vi "penaltyTactic.vi"(7 "firstCall":bool=TRUE, 8 "error in (no error)":errorcluster, 9 "Game in":refnum<class "Game.lvclass">, 10 "RobotRef":refnum<class "Robot.lvclass">, 11 "PenaltyTactic in":refnum<class "PenaltyTactic.lvclass">) -> (0 "error out":errorcluster, 2 "Robot out":refnum<class "Robot.lvclass">, 3 "PenaltyTactic out":refnum<class "PenaltyTactic.lvclass">)   [LabVIEW 2024, in "PenaltyTactic.lvclass"]
uses:
  PenaltyTactic.lvclass
  C:/Users/as119/OneDrive/Documentos/roboIME/SSL_AI/Tactic_class/Tactic.lvclass
  Robot_class/Robot.lvclass
  C:/Users/as119/OneDrive/Documentos/roboIME/SSL_AI/Object_class/Object.lvclass
  Game_class/Game.lvclass
  Robot_class/tactics.ctl
  Control 2.ctl
  Tactic_class/Tactic.lvclass/Tactic.ctl
  Game_class/Game.lvclass/Game.ctl
  Parameters_class/Parameters.lvclass/Parameters.ctl
  Team_class/Team.lvclass/Team.ctl
  Referee_class/Referee.lvclass/Referee.ctl
  Object_class/Object.lvclass/Object.ctl
  Skillbook_class/Skillbook.lvclass/Skillbook.ctl
  Robot_class/Robot.lvclass/Robot.ctl
  Robot_class/robotKickToStates.ctl
  Events_class/Events.lvclass/Events.ctl
  Ball_class/Ball.lvclass/Ball.ctl
  PenaltyTactic.lvclass/PenaltyTactic.ctl
  <vilib>/numeric/Random Number (Range) U64.vi
  Parameters_class/Read ShootOutForce.vi
  Game_class/Read FieldRef.vi
  Game_class/Read BallRef.vi
  Game_class/Read Parameters.lvclass.vi
  Game_class/Read NewParameters.vi
  Object_class/Read x.vi
  Skillbook_class/Read KickToSkill.vi
  Robot_class/Write kick_x.vi
  <vilib>/numeric/Random Number (Range) I64.vi
  Object_class/Read y.vi
  Object_class/Read position(x,y).vi
  Robot_class/Read robotKickState.vi
  Game_class/Read EventsRef.vi
  Events_class/Read kick.vi
  Ball_class/Read velocityNorm.vi
  Skillbook_class/Read HaltSkill.vi
  Game_class/Read EnemyRef.vi
  Game_class/Read Referee.vi
  Referee_class/Read enemy_goalie_id.vi
  Team_class/Read RobotRef.vi
  Parameters_class/Read KickForce.vi
  Parameters_class/Read AttakingOurselves.vi
  Parameters_class/Read KickAngle.vi
  Tactic_class/Read Skillbook.vi
  Robot_class/Write tactic.vi
  Write States.vi
  <vilib>/numeric/sub_Random U32.vi
  <vilib>/Analysis/_algsub.llb/Vector Norm.vi
  <vilib>/Analysis/_algsub.llb/Real Vector Norm.vi
  Enemy_class/Enemy.lvclass
  C:/Users/as119/OneDrive/Documentos/roboIME/SSL_AI/Team_class/Team.lvclass
  Ball_class/Ball.lvclass
  Parameters_class/Parameters.lvclass
  Referee_class/Referee.lvclass
  Skillbook_class/Skillbook.lvclass
  Field_class/Field.lvclass
  KickToSkill_class/KickToSkill.lvclass
  Events_class/Events.lvclass
  HaltSkill_class/HaltSkill.lvclass
  Utilities_class/Utilities.lvclass
  ShootTactic_class/ShootTactic.lvclass
panel:
  out "kick_x":dbl
  in  "factor goal width":dbl=0.75 format="%#_13g"
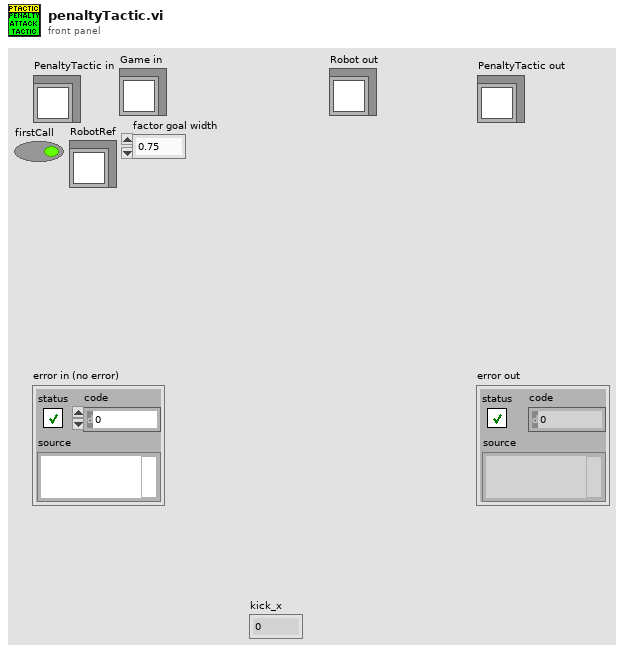
[diagram p1: front panel]
types:
  T1 = typedef "Control 2.ctl" = enum16{"Gotoball", "Kick", "Fake kick", "Position", "Exit"}
  T2 = typedef "tactics.ctl" = enum16{"GoToBallPlacementPosition", "PlaceBall", "GoToBallPlacement", "5Robots", "BallPlacementEnemy", "ReceivePassInFuturePoint", "Roller", "PrepareRollToPassRollerGoTo", "PrepareRollToPassReceiverGoTo", "WaitRoll", "PositionToRoll", "PenaltyAttacker", "PassObserver", "PenaltyDefense", "TableReceiverTactic", "Test", "DefendGoal", "Marker", "FollowAttacker", "DefendArea", "Shoot", "AttackerAimGoal", "AttackerBallOutOfField", "AttackerBlock", "AttackerStop", "Duelist", "Halt", "ZigZag", "GoTo", "Timeout", "KickToBestRobot", "KickToPassReceiver", "PositionToReceivePass", "WaitPass", "GoToTarget"}
  T3 = typedef "Control 2.ctl" = enum16{"Penalty", "Kick", "Pos3", "Pos2", "Pos1", "Exit"}
  T4 = typedef "robotKickToStates.ctl" = enum16{"shootFromDirect", "avoidCollideBall", "goToBackBall", "none", "walk", "turn", "turnAntiClockWise", "turnClockwise", "oldKickToShoot", "oldKickToGoToBackBall", "shoot"}
  T5 = typedef "NewParameters.ctl" = cluster{"PenaltyDistance":dbl, "DistanceAttackerToBackBall":dbl, "Division":enum16{"Div B", "Div A"}, "DistanceToAvoidyEnemyRobot":dbl, "BallPlacementDistance":dbl, "DisatanceBehindBallToStealBall":dbl, "MaxDistanceToPositionKickoff":dbl, "BlockEnemyTarget":bool, "MaxStopVAng":dbl, "DistanceMarkerToEnemy":dbl, "IgnoreDribblerContact":bool, "DistanceToBeginEnemyPosession":dbl, "GoToBallWhenEnemyNotMoving":bool, "EnemyDistanceToReduceVelocity":dbl, "TurnOnEnemyDistanceToReduceVelocity":bool, "EnemyDistanceToShootOutBall":dbl, "DefenseKickBall":bool, "MoreKickToGoal? (0-0.3)":dbl, "ChipKickInEnemyField":bool, "ShootOutRobotId":dbl, "FieldLenghtDenominatorInShootOut":dbl, "AdjustPositionInBallPlacement":bool, "PowerGodPass":dbl, "VelocityAbortEnemyPos":dbl, "MaxDistToBeginPass":dbl, "MinDistToBeginPass":dbl, "VelocityInDirects":dbl, "BadDribblerIDs":i32[], "NewKickToDistanceAroundBall":dbl, "PowerAvoidColisionMarker":dbl, "DistanceToAvoidColisionMarker":dbl, "AvoidBallKick":dbl, "DistanceTryKick":dbl, "SuicideKickDIstance":dbl, "AdjustFirstKickDistance":dbl, "AvoidAimLessKick":dbl, "DistanceToAvoidyEnemyShootRobot ":dbl, "NumberOfMarkers":dbl, "PotField":bool, "PIDLateral":bool, "MinDistanceFirstKickX":dbl, "MinDistanceFirstKickY":dbl, "FractionOfDistToTouchGround\nAfterChipKick":dbl, "FractionOfKickxWhen\nComposedWithKickz":dbl, "Style":T6, "MoveInTurnState":bool, "DistFromEnemyToConsider\nMoveInTurnState":dbl, "CascadePID":bool, "TurnAroundParameters":cluster{"Radius":dbl, "Multiplier":dbl, "ChordAngle":dbl}, "SafeDriveVel":dbl, "DistanceToGoToBackBall":dbl, "minDistanceToNotFinish\nEnemyPossession":dbl, "OneTouchShot":cluster{"angleFactor":dbl, "maxAngle":dbl, "Attack":bool, "Defense":bool}, "OpenAngleToGoal":cluster{"minAngle":dbl, "maxAngle":dbl, "minEvaluation":dbl}, "ShotInterception":cluster{"shotSpeed":dbl, "minEnemySpeed":dbl, "maxEnemySpeed":dbl, "minEvaluation":dbl}, "AllyTeamArray":T7[], "maxDefendersNumber":i32, "Zone":cluster{"GuardPositionArray":dbl[][], "ZoneMidField":dbl[], "CenterForwardWidth":dbl}, "MinEvaluationToShoot":dbl, "PassInterception":cluster{"maxPassSpeed":dbl, "minPassSpeed":dbl, "minEnemySpeed":dbl, "chipPassDistance":dbl, "chipPassEvaluation":dbl, "minEvaluation":dbl, "maxEnemySpeed":dbl}, "PassDistance":cluster{"maxDistance":dbl, "minDistance":dbl}, "receiverSpeed":dbl, "maxBallSpeed":dbl, "slackTime":dbl, "Turning radius":dbl, "Turning v_ang":dbl, "AlignError":cluster{"Distance":dbl, "Orientation":dbl, "V_norm(m/s)":dbl, "V_ang (rad/s)":dbl}, "RobotRadius":dbl, "KickerDistance":dbl, "keeper angle  to cover goalpost":dbl, "a_slide":dbl, "a_roll":dbl, "k_switch":dbl, "Penalty":u16}
  T6 = typedef "Style.ctl" = enum16{"Insanity", "Offensive", "Defensive"}
  T7 = typedef "AllyTeam.ctl" = enum16{"Keeper", "Defender", "Attacker"}
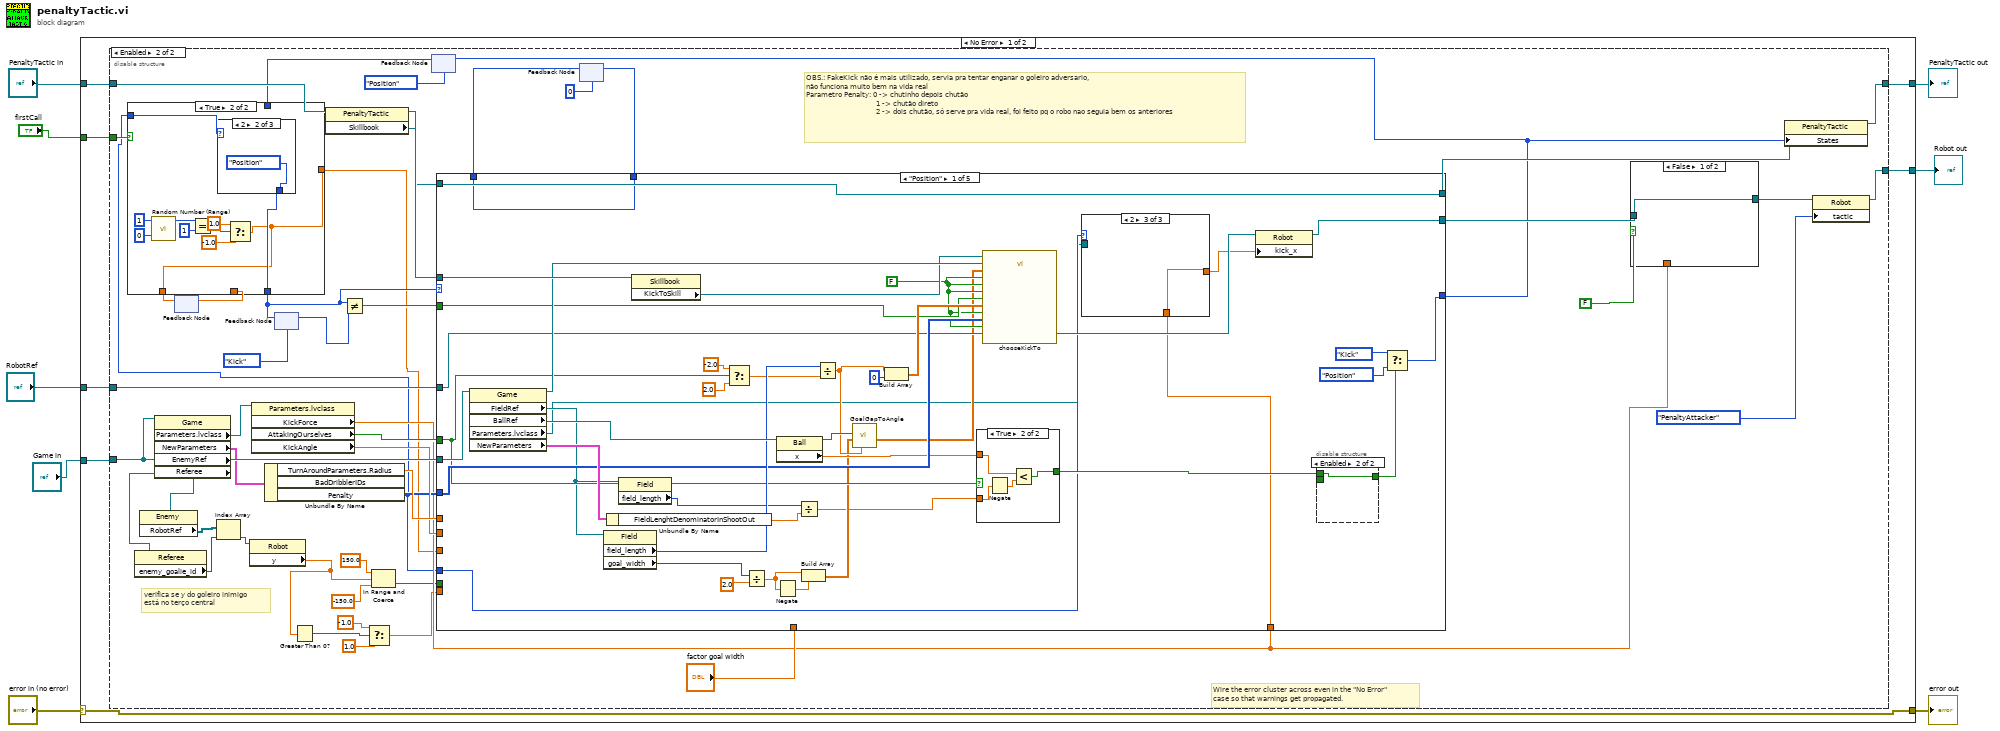
[diagram p0: block diagram]
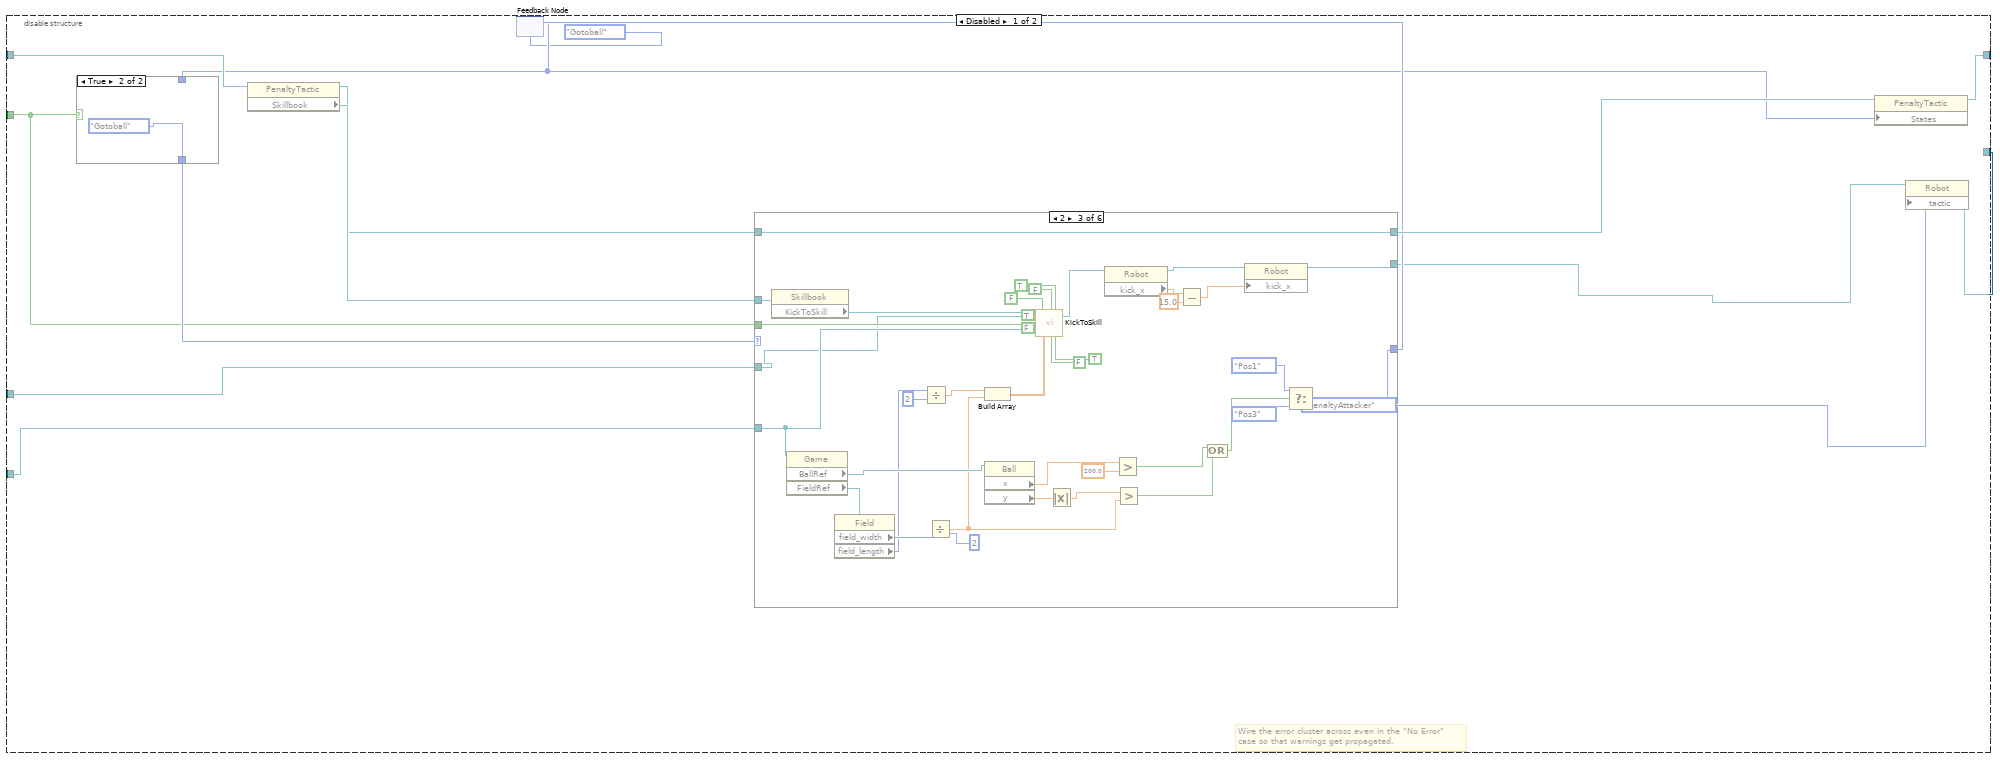
[diagram p2: hidden frame]
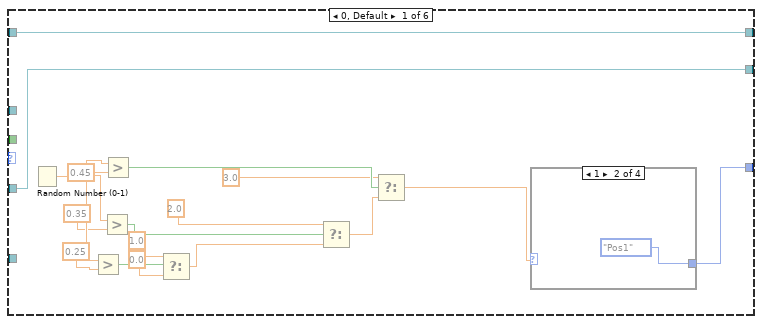
[diagram p3: hidden frame]
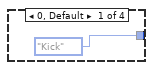
[diagram p4: hidden frame]
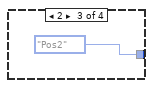
[diagram p5: hidden frame]
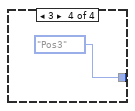
[diagram p6: hidden frame]
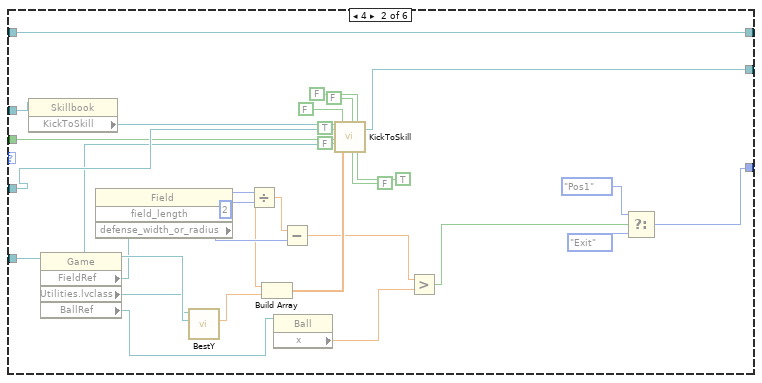
[diagram p7: hidden frame]
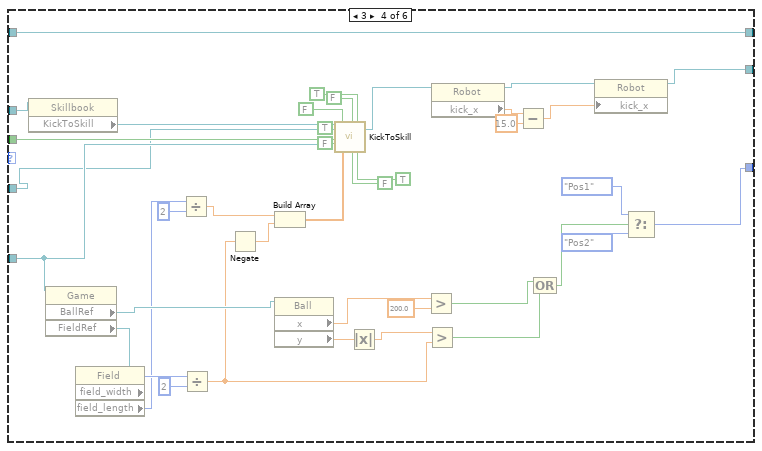
[diagram p8: hidden frame]
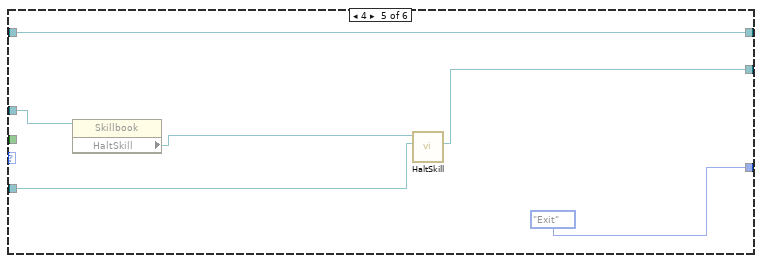
[diagram p9: hidden frame]
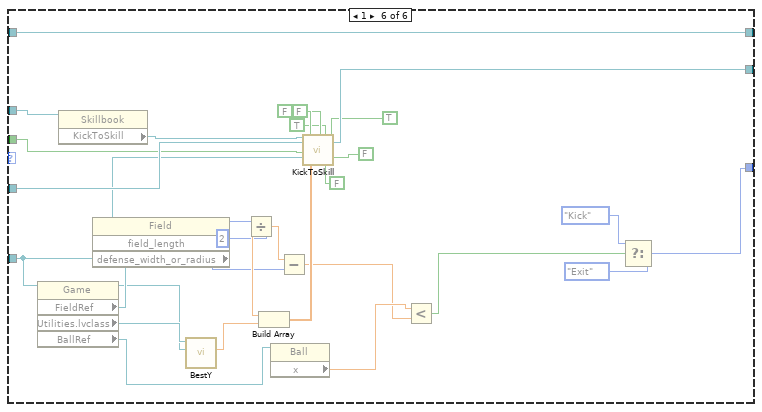
[diagram p10: hidden frame]
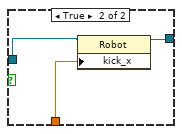
[diagram p12: hidden frame]
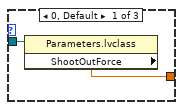
[diagram p13: hidden frame]
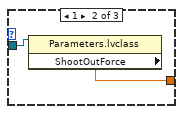
[diagram p14: hidden frame]
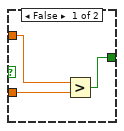
[diagram p15: hidden frame]
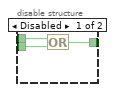
[diagram p16: hidden frame]
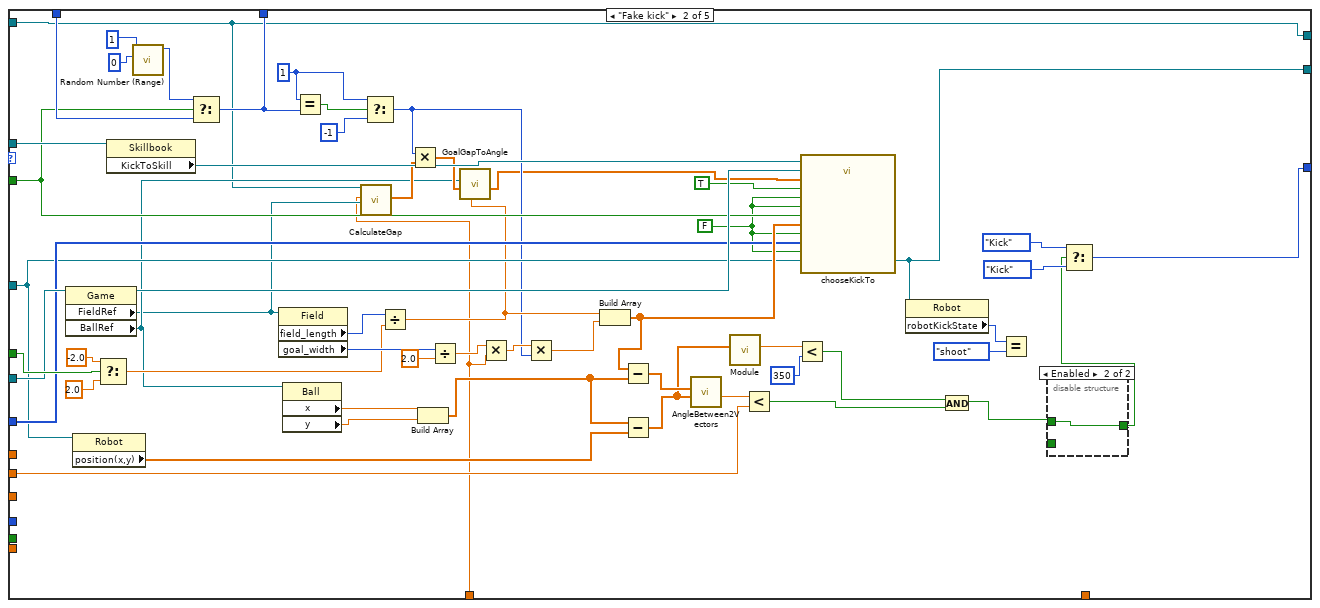
[diagram p17: hidden frame]
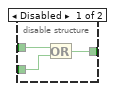
[diagram p18: hidden frame]
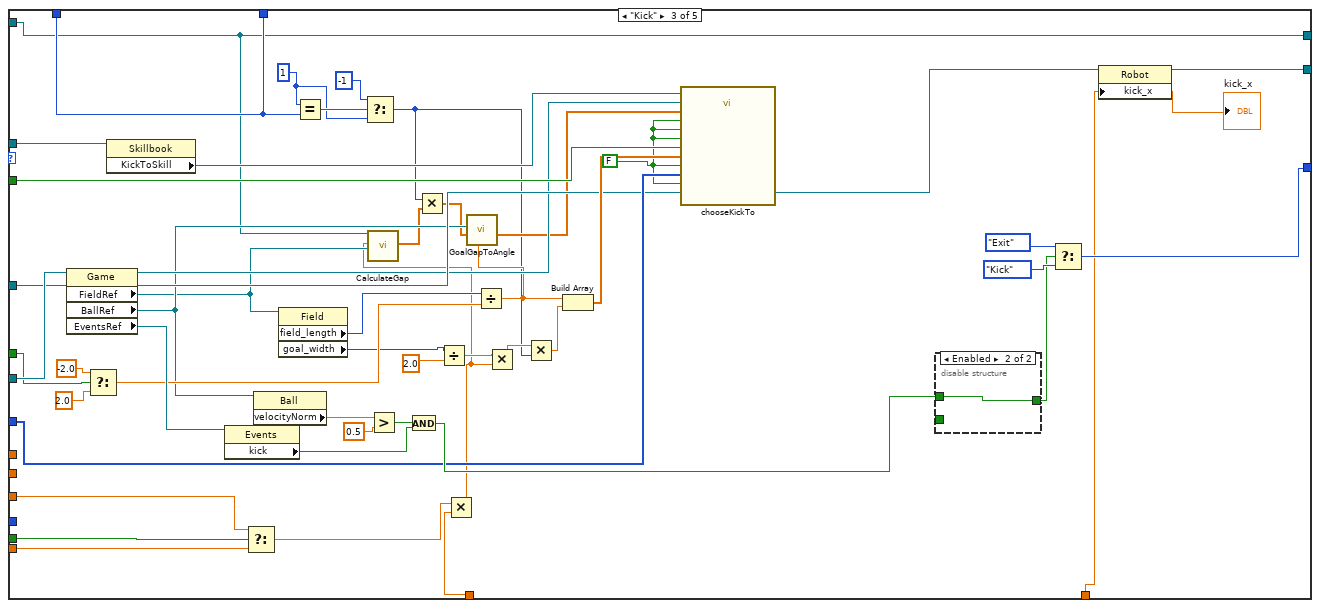
[diagram p19: hidden frame]
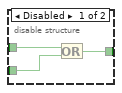
[diagram p20: hidden frame]
diagram:
  n1 = case shown="No Error" "error in (no error)" {
    selector: "error in (no error)" -> [w15 w450]
    tunnel: [w15 w450] -> w7
    tunnel: [w13 w449] -> w5
    tunnel: "PenaltyTactic in" -> [w14 w449]
    tunnel: "firstCall" -> [w9 _]
    tunnel: [w12 w448] -> w3
    tunnel: "RobotRef" -> [w11 w448]
    tunnel: "Game in" -> [w10 _]
    frame No Error {
      n2 = disable-structure shown="Enabled" {
        disable-tunnel: w14 -> [w29 w243]
        disable-tunnel: [w25 w239] -> w13
        disable-tunnel: [w24 w238] -> w12
        disable-tunnel: w11 -> [w23 w237]
        disable-tunnel: w10 -> [w18 w222]
        disable-tunnel: w9 -> [w16 w233]
        frame Disabled {
          # "Wire the error cluster across even in the \"No Error\"\ncase so that warnings get propagated."
          n3 = property class="PenaltyTactic"(reference=w29) -> (reference out=w27:refnum<class "PenaltyTactic.lvclass">, "Skillbook"=w28:refnum<class "Skillbook.lvclass">)  [unwired: 1 in, 1 out]
          n4 = feedback #1(Control_2."Gotoball" ("States")) -> (w20:u16)
          n5 = case shown="True" w16 {
            tunnel: [w194 Control_2."Gotoball" ("States")] -> w30
            tunnel: w20 -> [w194 _]
            frame False {
            }
            frame True {
            }
          }
          n6 = case shown="2" w30 {
            tunnel: w28 -> [_ w78 w116 w155 w162 w192]
            tunnel: [w32 w77 w115 w154 w164 w193] -> w26
            tunnel: w27 -> [w32 w77 w115 w154 w164 w193]
            tunnel: w23 -> [w31 w75 w105 w144 w160 w190]
            tunnel: [w33 w79 w117 w156 Control_2."Exit" ("States") w172] -> w21
            tunnel: w18 -> [_ w67 w107 w146 _ w169]
            tunnel: [w31 w73 w91 w125 w159 w188] -> w17
            tunnel: w16 -> [_ w74 w113 w152 _ w189]
            frame 0, Default {
              n7 = Random Number (0-1)() -> (number: 0 to 1=w47:dbl)
              n8 = Greater?(x=w47, y=0.25) -> (0:w43:bool)
              n9 = Greater?(x=w47, y=0.35) -> (0:w39:bool)
              n10 = Greater?(x=w47, y=0.45) -> (0:w36:bool)
              n11 = Select(t=1.0, s=w43, f=0.0) -> (s? t:f=w40:dbl)
              n12 = Select(t=2.0, s=w39, f=w40) -> (s? t:f=w37:dbl)
              n13 = Select(t=3.0, s=w36, f=w37) -> (s? t:f=w34:dbl)
              n14 = case shown="1" w34 {
                tunnel: [Control_2."Kick" ("States") Control_2."Pos1" ("States") Control_2."Pos2" ("States") Control_2."Pos3" ("States")] -> w33
                frame 0, Default {
                }
                frame 1 {
                }
                frame 2 {
                }
                frame 3 {
                }
              }
            }
            frame 4 {
              n15 = property class="Skillbook"(reference=w78) -> ("KickToSkill"=w76:refnum<class "KickToSkill.lvclass">)  [unwired: 1 in, 2 out]
              n16 = property class="Game"(reference=w67) -> (reference out=w64:refnum<class "Game.lvclass">, "FieldRef"=w62:refnum<class "Field.lvclass">, "Utilities.lvclass"=w63:refnum<class "Utilities.lvclass">, "BallRef"=w57:refnum<class "Ball.lvclass">)  [unwired: 1 in, 1 out]
              n17 = property class="Field"(reference=w62) -> ("field_length"=w61:i32, "defense_width_or_radius"=w59:i32)  [unwired: 1 in, 2 out]
              n18 = call "BestY.vi"("Utilities in"=w63, "Game"=w64) -> ("Best y"=w65:dbl)  [unwired: 3 in, 4 out]
              n19 = Divide(x=w61, y=2) -> (x/y=w58:dbl)
              n20 = Build Array(w58, w65) -> (w66:dbl[])
              n21 = property class="Ball"(reference=w57) -> ("x"=w56:dbl)  [unwired: 1 in, 2 out]
              n22 = Subtract(x=w58, y=w59) -> (x-y=w55:dbl)
              n23 = call "KickToSkill.vi"("KickToSkill in"=w76, "Robot"=w75, "firstCall?"=w74, "Game"=w67, "use criteria?"=FALSE, "Target"=w66, "chipKick ?"=FALSE, "KickForce 0?"=FALSE, "WeakKick"=FALSE, "ForceInGame"=TRUE, "IgnorePosEst"=TRUE, "pass?"=FALSE) -> ("Robot out"=w73:refnum<class "Robot.lvclass">)  [unwired: 4 in, 3 out]
              n24 = Greater?(x=w55, y=w56) -> (0:w54:bool)
              n25 = Select(t=Control_2."Pos1" ("States"), s=w54, f=Control_2."Exit" ("States")) -> (s? t:f=w79:u16)
            }
            frame 2 {
              n26 = property class="Skillbook"(reference=w116) -> ("KickToSkill"=w114:refnum<class "KickToSkill.lvclass">)  [unwired: 1 in, 2 out]
              n27 = property class="Game"(reference=w107) -> ("BallRef"=w106:refnum<class "Ball.lvclass">, "FieldRef"=w100:refnum<class "Field.lvclass">)  [unwired: 1 in, 2 out]
              n28 = property class="Field"(reference=w100) -> ("field_width"=w95:i32, "field_length"=w83:i32)  [unwired: 1 in, 2 out]
              n29 = Divide(x=w83, y=2) -> (x/y=w84:dbl)
              n30 = Divide(x=w95, y=2) -> (x/y=w82:dbl)
              n31 = Build Array(w84, w82) -> (w94:dbl[])
              n32 = property class="Ball"(reference=w106) -> ("x"=w104:dbl, "y"=w102:dbl)  [unwired: 1 in, 2 out]
              n33 = call "KickToSkill.vi"("KickToSkill in"=w114, "Robot"=w105, "firstCall?"=w113, "Game"=w107, "use criteria?"=FALSE, "Target"=w94, "chipKick ?"=FALSE, "KickForce 0?"=FALSE, "WeakKick"=TRUE, "ForceInGame"=TRUE, "IgnorePosEst"=TRUE, "pass?"=FALSE) -> ("Robot out"=w92:refnum<class "Robot.lvclass">)  [unwired: 4 in, 3 out]
              n34 = Absolute Value(x=w102) -> (abs(x)=w101:dbl)
              n35 = property class="Robot"(reference=w92) -> (reference out=w90:refnum<class "Robot.lvclass">, "kick_x"=w89:dbl)  [unwired: 1 in, 1 out]
              n36 = Greater?(x=w104, y=200.0) -> (0:w98:bool)
              n37 = Greater?(x=w101, y=w82) -> (0:w97:bool)
              n38 = Subtract(x=w89, y=15.0) -> (x-y=w88:dbl)
              n39 = Compound Arithmetic op=OR(w98, w97) -> (w96:bool)
              n40 = property class="Robot"(reference=w90, "kick_x"=w88) -> (reference out=w91:refnum<class "Robot.lvclass">)  [unwired: 1 in, 1 out]
              n41 = Select(t=Control_2."Pos1" ("States"), s=w96, f=Control_2."Pos3" ("States")) -> (s? t:f=w117:T3)
            }
            frame 3 {
              n42 = property class="Skillbook"(reference=w155) -> ("KickToSkill"=w153:refnum<class "KickToSkill.lvclass">)  [unwired: 1 in, 2 out]
              n43 = property class="Game"(reference=w146) -> ("BallRef"=w145:refnum<class "Ball.lvclass">, "FieldRef"=w139:refnum<class "Field.lvclass">)  [unwired: 1 in, 2 out]
              n44 = property class="Field"(reference=w139) -> ("field_width"=w133:i32, "field_length"=w122:i32)  [unwired: 1 in, 2 out]
              n45 = Divide(x=w122, y=2) -> (x/y=w123:dbl)
              n46 = Divide(x=w133, y=2) -> (x/y=w120:dbl)
              n47 = Negate(x=w120) -> (-x=w134:dbl)
              n48 = Build Array(w123, w134) -> (w132:dbl[])
              n49 = property class="Ball"(reference=w145) -> ("x"=w143:dbl, "y"=w141:dbl)  [unwired: 1 in, 2 out]
              n50 = call "KickToSkill.vi"("KickToSkill in"=w153, "Robot"=w144, "firstCall?"=w152, "Game"=w146, "use criteria?"=FALSE, "Target"=w132, "chipKick ?"=FALSE, "KickForce 0?"=FALSE, "WeakKick"=TRUE, "ForceInGame"=TRUE, "IgnorePosEst"=TRUE, "pass?"=FALSE) -> ("Robot out"=w126:refnum<class "Robot.lvclass">)  [unwired: 4 in, 3 out]
              n51 = Absolute Value(x=w141) -> (abs(x)=w140:dbl)
              n52 = Greater?(x=w143, y=200.0) -> (0:w137:bool)
              n53 = Greater?(x=w140, y=w120) -> (0:w136:bool)
              n54 = property class="Robot"(reference=w126) -> (reference out=w130:refnum<class "Robot.lvclass">, "kick_x"=w129:dbl)  [unwired: 1 in, 1 out]
              n55 = Subtract(x=w129, y=15.0) -> (x-y=w128:dbl)
              n56 = Compound Arithmetic op=OR(w137, w136) -> (w135:bool)
              n57 = property class="Robot"(reference=w130, "kick_x"=w128) -> (reference out=w125:refnum<class "Robot.lvclass">)  [unwired: 1 in, 1 out]
              n58 = Select(t=Control_2."Pos1" ("States"), s=w135, f=Control_2."Pos2" ("States")) -> (s? t:f=w156:T3)
            }
            frame 4 {
              n59 = property class="Skillbook"(reference=w162) -> ("HaltSkill"=w161:refnum<class "HaltSkill.lvclass">)  [unwired: 1 in, 2 out]
              n60 = call-dynamic "HaltSkill.vi"("Robot"=w160, "HaltSkill in"=w161) -> ("Robot out"=w159:refnum<class "Robot.lvclass">)  [unwired: 7 in, 2 out]
            }
            frame 1 {
              n61 = property class="Game"(reference=w169) -> (reference out=w176:refnum<class "Game.lvclass">, "FieldRef"=w178:refnum<class "Field.lvclass">, "Utilities.lvclass"=w177:refnum<class "Utilities.lvclass">, "BallRef"=w182:refnum<class "Ball.lvclass">)  [unwired: 1 in, 1 out]
              n62 = property class="Skillbook"(reference=w192) -> ("KickToSkill"=w191:refnum<class "KickToSkill.lvclass">)  [unwired: 1 in, 2 out]
              n63 = property class="Field"(reference=w178) -> ("field_length"=w179:i32, "defense_width_or_radius"=w180:i32)  [unwired: 1 in, 2 out]
              n64 = call "BestY.vi"("Utilities in"=w177, "Game"=w176) -> ("Best y"=w175:dbl)  [unwired: 3 in, 4 out]
              n65 = Divide(x=w179, y=2) -> (x/y=w181:dbl)
              n66 = Build Array(w181, w175) -> (w170:dbl[])
              n67 = property class="Ball"(reference=w182) -> ("x"=w167:dbl)  [unwired: 1 in, 2 out]
              n68 = Subtract(x=w181, y=w180) -> (x-y=w166:dbl)
              n69 = call "KickToSkill.vi"("KickToSkill in"=w191, "Robot"=w190, "firstCall?"=w189, "Game"=w169, "use criteria?"=FALSE, "Target"=w170, "chipKick ?"=FALSE, "WeakKick"=TRUE, "ForceInGame"=FALSE, "IgnorePosEst"=TRUE, "pass?"=FALSE) -> ("Robot out"=w188:refnum<class "Robot.lvclass">)  [unwired: 5 in, 3 out]
              n70 = Less?(x=w167, y=w166) -> (x < y?=w183:bool)
              n71 = Select(t=Control_2."Kick" ("States"), s=w183, f=Control_2."Exit" ("States")) -> (s? t:f=w172:T1)
            }
          }
          n72 = feedback-in #1(w21) -> ()
          n73 = property class="PenaltyTactic"(reference=w26, "States"=w20) -> (reference out=w25:refnum<class "PenaltyTactic.lvclass">)  [unwired: 1 in, 1 out]
          n74 = property class="Robot"(reference=w17, "tactic"=tactics."PenaltyAttacker") -> (reference out=w24:refnum<class "Robot.lvclass">)  [unwired: 1 in, 1 out]
        }
        frame Enabled {
          # "OBS.: FakeKick não é mais utilizado, servia pra tentar enganar o goleiro adversario, \nnão funciona muito bem na vida real\nParametro Penalty: 0 -> chutinho depois chutão\n                                   1 -> chutão direto\n                                   2 -> dois chutão, só serve pra vida real, foi feito pq o robo nao seguia bem os anteriores"
          # "verifica se y do goleiro inimigo\nestá no terço central"
          # "Wire the error cluster across even in the \"No Error\"\ncase so that warnings get propagated."
          n75 = property class="Game"(reference=w222) -> ("Parameters.lvclass"=w221:refnum<class "Parameters.lvclass">, "NewParameters"=w218:T5, "EnemyRef"=w209:refnum<class "Enemy.lvclass">, "Referee"=w208:refnum<class "Referee.lvclass">)  [unwired: 1 in, 2 out]
          n76 = property class="Referee"(reference=w208) -> ("enemy_goalie_id"=w206:i32)  [unwired: 1 in, 2 out]
          n77 = property class="Enemy"(reference=w209) -> ("RobotRef"=w207:refnum<class "Robot.lvclass">[])  [unwired: 1 in, 2 out]
          n78 = feedback #2() -> (w210:dbl)  [unwired: 1 in]
          n79 = Index Array(array=w207, index=w206) -> (element=w205:refnum<class "Robot.lvclass">)
          n80 = property class="Robot"(reference=w205) -> ("y"=w198:dbl)  [unwired: 1 in, 2 out]
          n81 = property class="Parameters.lvclass"(reference=w221) -> ("KickForce"=w213:dbl, "AttakingOurselves"=w220:bool, "KickAngle"=w216:dbl)  [unwired: 1 in, 2 out]
          n82 = Unbundle By Name(w218) -> ("TurnAroundParameters.Radius"=w217:dbl, "BadDribblerIDs"=w215:i32[], "Penalty"=w196:u16)
          n83 = feedback #3(Control_2."Kick" ("States")) -> (w229:T1)
          n84 = Greater Than 0?(x=w198) -> (x > 0?=w201:bool)
          n85 = property class="PenaltyTactic"(reference=w243) -> (reference out=w241:refnum<class "PenaltyTactic.lvclass">, "Skillbook"=w242:refnum<class "Skillbook.lvclass">)  [unwired: 1 in, 1 out]
          n86 = Select(t=-1.0, s=w201, f=1.0) -> (s? t:f=w197:dbl)
          n87 = In Range and Coerce(upper limit=150.0 ("x"), x=w198, lower limit=-150.0 ("x")) -> (In Range?=w202:bool)  [unwired: 1 out]
          n88 = feedback #4(Control_2."Position" ("States")) -> (w235:T1)
          n89 = case shown="True" w233 {
            tunnel: [w434 w444] -> w227
            tunnel: w235 -> [w434 _]
            tunnel: [w433 w436] -> w212
            tunnel: [w433 w436] -> w211
            tunnel: w210 -> [w433 _]
            tunnel: w196 -> [_ w435]
            frame False {
            }
            frame True {
              n90 = call-poly <vilib>:"Random Number (Range).vi"("lower bound (0)"=u64 0, "upper bound (100)"=u64 1) -> ("number"=w441:u64)  [unwired: 9 in]
              n91 = Equal?(x=w441, y=u64 1) -> (x = y?=w439:bool)
              n92 = case shown="2" w435 {
                tunnel: [Control_2."Position" ("States") Control_2."Position" ("States") Control_2."Kick" ("States")] -> w444
                frame 0, Default {
                }
                frame 2 {
                }
                frame 1 {
                }
              }
              n93 = Select(t=1.0, s=w439, f=-1.0) -> (s? t:f=w436:dbl)
            }
          }
          n94 = feedback-in #2(w211) -> ()
          n95 = feedback-in #3(w227) -> ()
          n96 = Not Equal?(x=w227, y=w229) -> (x != y?=w226:bool)
          n97 = feedback #5(0) -> (w223:i64)
          n98 = case shown="\"Position\"" w227 {
            selector: w227 -> [_ _ _ _ w430]
            tunnel: w242 -> [w289 w362 w416 w426 _]
            tunnel: [w288 w314 w378 w428 w432] -> w240
            tunnel: w241 -> [w288 w314 w378 w428 w432]
            tunnel: w237 -> [w269 w324 w391 w424 w431]
            tunnel: [w283 w360 w413 Control_2."Exit" ("States") w430] -> w230
            tunnel: w222 -> [w287 w339 w415 _ _]
            tunnel: [w275 w322 w395 w423 w431] -> w231
            tunnel: w226 -> [w271 w328 w390 _ _]
            tunnel: [w279 w350 w396 w422 w429] -> w224
            tunnel: w223 -> [w279 w355 w396 w422 w429]
            tunnel: w220 -> [w265 w340 w400 _ _]
            tunnel: "factor goal width" -> [_ w312 w373 _ _]
            tunnel: w217 -> [_ _ _ _ _]
            tunnel: w216 -> [_ w332 _ _ _]
            tunnel: w215 -> [w270 w326 w394 _ _]
            tunnel: w213 -> [w248 _ w374 _ _]
            tunnel: w212 -> [_ _ w370 _ _]
            tunnel: w202 -> [_ _ w371 _ _]
            tunnel: w197 -> [_ _ w369 _ _]
            tunnel: w196 -> [w251 _ _ _ _]
            frame "Position" {
              w267 = FALSE ("ForceInGame")
              n99 = property class="Game"(reference=w287) -> (reference out=w273:refnum<class "Game.lvclass">, "FieldRef"=w255:refnum<class "Field.lvclass">, "BallRef"=w286:refnum<class "Ball.lvclass">, "Parameters.lvclass"=w250:refnum<class "Parameters.lvclass">, "NewParameters"=w285:T5)  [unwired: 1 in, 1 out]
              n100 = property class="Field"(reference=w255) -> ("field_length"=w282:i32, "goal_width"=w260:i32)  [unwired: 1 in, 2 out]
              n101 = Unbundle By Name(w285) -> ("FieldLenghtDenominatorInShootOut"=w253:dbl)
              n102 = property class="Field"(reference=w255) -> ("field_length"=w254:i32)  [unwired: 1 in, 2 out]
              n103 = property class="Skillbook"(reference=w289) -> ("KickToSkill"=w272:refnum<class "KickToSkill.lvclass">)  [unwired: 1 in, 2 out]
              n104 = Select(t=-2.0, s=w265, f=2.0 ("y")) -> (s? t:f=w276:dbl)
              n105 = Divide(x=w260, y=2.0) -> (x/y=w258:dbl)
              n106 = Negate(x=w258) -> (-x=w257:dbl)
              n107 = property class="Ball"(reference=w286) -> (reference out=w262:refnum<class "Ball.lvclass">, "x"=w264:dbl)  [unwired: 1 in, 1 out]
              n108 = Divide(x=w254, y=w253) -> (x/y=w252:dbl)
              n109 = Build Array(w258, w257) -> (w256:dbl[])
              n110 = Divide(x=w282, y=w276) -> (x/y=w261:dbl)
              n111 = call "GoalGapToAngle.vi"("x_goal"=w261, "GoalGap"=w256, "Ball"=w262) -> ("angle gap"=w263:dbl[])  [unwired: 6 in, 2 out]
              n112 = Build Array(w261, 0) -> (w274:dbl[])
              n113 = case shown="True" w265 {
                tunnel: w252 -> [w298 w300]
                tunnel: [w297 w302] -> w266
                tunnel: w264 -> [w296 w301]
                frame False {
                  n114 = Greater?(x=w296, y=w298) -> (0:w297:bool)
                }
                frame True {
                  n115 = Negate(x=w300) -> (-x=w299:dbl)
                  n116 = Less?(x=w301, y=w299) -> (x < y?=w302:bool)
                }
              }
              n117 = call "chooseKickTo.vi"("KickToSkill in"=w272, "Game in"=w273, "target gap"=w263, "Robot"=w269, "KickForce 0?"=w267, "use criteria?"=w267, "ForceInGame"=w267, "BadDribblerIDs"=w270, "pass?"=w267, "firstCall"=w271, "ChipKickInEnemyField"=w267, "Target"=w274) -> ("Robot out"=w268:refnum<class "Robot.lvclass">)  [unwired: 14 in, 1 out]
              n118 = case shown="2" w251 {
                tunnel: w250 -> [w292 w294 _]
                tunnel: [w291 w293 w295] -> w249
                tunnel: w248 -> [_ _ w295]
                frame 0, Default {
                  n119 = property class="Parameters.lvclass"(reference=w292) -> ("ShootOutForce"=w291:dbl)  [unwired: 1 in, 2 out]
                }
                frame 1 {
                  n120 = property class="Parameters.lvclass"(reference=w294) -> ("ShootOutForce"=w293:dbl)  [unwired: 1 in, 2 out]
                }
                frame 2 {
                }
              }
              n121 = property class="Robot"(reference=w268, "kick_x"=w249) -> (reference out=w275:refnum<class "Robot.lvclass">)  [unwired: 1 in, 1 out]
              n122 = disable-structure shown="Enabled" {
                disable-tunnel: [w305 w306] -> w280
                disable-tunnel: w266 -> [w304 w306]
                disable-tunnel: _ -> [w303 _]
                frame Disabled {
                  n123 = Or(x=w304, y=w303) -> (x .or. y?=w305:bool)
                }
                frame Enabled {
                }
              }
              n124 = Select(t=Control_2."Kick" ("States"), s=w280, f=Control_2."Position" ("States")) -> (s? t:f=w283:T1)
            }
            frame "Fake kick" {
              w325 = FALSE
              w351 = 1
              n125 = property class="Game"(reference=w339) -> (reference out=w330:refnum<class "Game.lvclass">, "FieldRef"=w315:refnum<class "Field.lvclass">, "BallRef"=w316:refnum<class "Ball.lvclass">)  [unwired: 1 in, 1 out]
              n126 = property class="Robot"(reference=w324) -> ("position(x,y)"=w344:dbl[])  [unwired: 1 in, 2 out]
              n127 = Select(t=-2.0, s=w340, f=2.0 ("y")) -> (s? t:f=w323:dbl)
              n128 = property class="Skillbook"(reference=w362) -> ("KickToSkill"=w331:refnum<class "KickToSkill.lvclass">)  [unwired: 1 in, 2 out]
              n129 = call-poly <vilib>:"Random Number (Range).vi"("lower bound (-100)"=0, "upper bound (100)"=1) -> ("number"=w358:i64)  [unwired: 9 in]
              n130 = Select(t=w358, s=w328, f=w355) -> (s? t:f=w350:i64)
              n131 = property class="Field"(reference=w315) -> ("field_length"=w359:i32, "goal_width"=w354:i32)  [unwired: 1 in, 2 out]
              n132 = property class="Ball"(reference=w316) -> ("x"=w348:dbl, "y"=w347:dbl)  [unwired: 1 in, 2 out]
              n133 = Equal?(x=w351, y=w350) -> (x = y?=w349:bool)
              n134 = call-dynamic "CalculateGap.vi"("object in"=w314, "factor"=w312, "FieldRef"=w315) -> ("gap"=w319:dbl[])  [unwired: 14 in, 2 out]
              n135 = Select(t=w351, s=w349, f=-1) -> (s? t:f=w310:i32)
              n136 = Divide(x=w359, y=w323) -> (x/y=w317:dbl)
              n137 = Multiply(x=w310, y=w319) -> (x*y=w318:dbl[])
              n138 = Build Array(w348, w347) -> (w345:dbl[])
              n139 = Divide(x=w354, y=2.0) -> (x/y=w313:dbl)
              n140 = call "GoalGapToAngle.vi"("x_goal"=w317, "GoalGap"=w318, "Ball"=w316) -> ("angle gap"=w309:dbl[])  [unwired: 6 in, 2 out]
              n141 = Multiply(x=w313, y=w312) -> (x*y=w311:dbl)
              n142 = Multiply(x=w311, y=w310) -> (x*y=w353:dbl)
              n143 = Build Array(w317, w353) -> (w327:dbl[])
              n144 = Subtract(x=w327, y=w345) -> (x-y=w346:dbl[])
              n145 = Subtract(x=w345, y=w344) -> (x-y=w333:dbl[])
              n146 = call "AngleBetween2Vectors.vi"("Array 1"=w333, "Array 2"=w346) -> ("angleInDegrees"=w343:dbl)  [unwired: 6 in, 3 out]
              n147 = call "Module.vi"("2D vector"=w333) -> ("Modulo"=w336:dbl)  [unwired: 8 in, 2 out]
              n148 = Less?(x=w343, y=w332) -> (x < y?=w338:bool)
              n149 = Less?(x=w336, y=350) -> (x < y?=w335:bool)
              n150 = call "chooseKickTo.vi"("KickToSkill in"=w331, "Game in"=w330, "target gap"=w309, "Robot"=w324, "KickForce 0?"=TRUE, "use criteria?"=w325, "ForceInGame"=w325, "BadDribblerIDs"=w326, "pass?"=w325, "firstCall"=w328, "ChipKickInEnemyField"=w325, "Target"=w327) -> ("Robot out"=w322:refnum<class "Robot.lvclass">)  [unwired: 14 in, 1 out]
              n151 = property class="Robot"(reference=w322) -> ("robotKickState"=w321:T4)  [unwired: 1 in, 2 out]
              n152 = And(x=w335, y=w338) -> (x .and. y?=w337:bool)
              n153 = Equal?(x=w321, y=robotKickToStates."shoot") -> ()  [unwired: 1 out]
              n154 = disable-structure shown="Enabled" {
                disable-tunnel: [w366 w367] -> w307
                disable-tunnel: _ -> [w365 _]
                disable-tunnel: w337 -> [w364 w367]
                frame Disabled {
                  n155 = Or(x=w364, y=w365) -> (x .or. y?=w366:bool)
                }
                frame Enabled {
                }
              }
              n156 = Select(t=Control_2."Kick" ("States"), s=w307, f=Control_2."Kick" ("States")) -> (s? t:f=w360:T1)
            }
            frame "Kick" {
              w389 = FALSE ("ChipKickInEnemyField")
              w398 = 1
              n157 = property class="Game"(reference=w415) -> (reference out=w388:refnum<class "Game.lvclass">, "FieldRef"=w379:refnum<class "Field.lvclass">, "BallRef"=w384:refnum<class "Ball.lvclass">, "EventsRef"=w408:refnum<class "Events.lvclass">)  [unwired: 1 in, 1 out]
              n158 = Select(t=-2.0, s=w400, f=2.0 ("y")) -> (s? t:f=w399:dbl)
              n159 = property class="Skillbook"(reference=w416) -> ("KickToSkill"=w393:refnum<class "KickToSkill.lvclass">)  [unwired: 1 in, 2 out]
              n160 = property class="Events"(reference=w408) -> ("kick"=w407:bool)  [unwired: 1 in, 2 out]
              n161 = Select(t=w370, s=w371, f=w369) -> (s? t:f=w368:dbl)
              n162 = property class="Ball"(reference=w384) -> ("velocityNorm"=w406:dbl)  [unwired: 1 in, 2 out]
              n163 = property class="Field"(reference=w379) -> ("field_length"=w412:i32, "goal_width"=w383:i32)  [unwired: 1 in, 2 out]
              n164 = Equal?(x=w398, y=w396) -> (x = y?=w409:bool)
              n165 = Select(t=-1, s=w409, f=w398) -> (s? t:f=w376:i32)
              n166 = Greater?(x=w406, y=0.5) -> (0:w404:bool)
              n167 = And(x=w404, y=w407) -> (x .and. y?=w403:bool)
              n168 = Divide(x=w383, y=2.0) -> (x/y=w380:dbl)
              n169 = Multiply(x=w368, y=w373) -> (x*y=w372:dbl)
              n170 = call-dynamic "CalculateGap.vi"("object in"=w378, "factor"=w372, "FieldRef"=w379) -> ("gap"=w377:dbl[])  [unwired: 14 in, 2 out]
              n171 = Multiply(x=w376, y=w377) -> (x*y=w375:dbl[])
              n172 = Divide(x=w412, y=w399) -> (x/y=w385:dbl)
              n173 = call "GoalGapToAngle.vi"("x_goal"=w385, "GoalGap"=w375, "Ball"=w384) -> ("angle gap"=w386:dbl[])  [unwired: 6 in, 2 out]
              n174 = Multiply(x=w380, y=w372) -> (x*y=w381:dbl)
              n175 = Multiply(x=w381, y=w376) -> (x*y=w410:dbl)
              n176 = Build Array(w385, w410) -> (w392:dbl[])
              n177 = call "chooseKickTo.vi"("KickToSkill in"=w393, "Game in"=w388, "target gap"=w386, "Robot"=w391, "KickForce 0?"=w389, "use criteria?"=w389, "ForceInGame"=w389, "BadDribblerIDs"=w394, "pass?"=w389, "firstCall"=w390, "ChipKickInEnemyField"=w389, "Target"=w392) -> ("Robot out"=w387:refnum<class "Robot.lvclass">)  [unwired: 14 in, 1 out]
              n178 = disable-structure shown="Enabled" {
                disable-tunnel: [w420 w421] -> w411
                disable-tunnel: _ -> [w419 _]
                disable-tunnel: w403 -> [w418 w421]
                frame Disabled {
                  n179 = Or(x=w418, y=w419) -> (x .or. y?=w420:bool)
                }
                frame Enabled {
                }
              }
              n180 = Select(t=Control_2."Exit" ("States"), s=w411, f=Control_2."Kick" ("States")) -> (s? t:f=w413:T1)
              n181 = property class="Robot"(reference=w387, "kick_x"=w374) -> (reference out=w395:refnum<class "Robot.lvclass">)  [unwired: 1 in, 1 out]
              "kick_x" <- w374
            }
            frame "Exit" {
              n182 = property class="Skillbook"(reference=w426) -> ("HaltSkill"=w425:refnum<class "HaltSkill.lvclass">)  [unwired: 1 in, 2 out]
              n183 = call-dynamic "HaltSkill.vi"("Robot"=w424, "HaltSkill in"=w425) -> ("Robot out"=w423:refnum<class "Robot.lvclass">)  [unwired: 7 in, 2 out]
            }
            frame "Gotoball" {
            }
          }
          n184 = feedback-in #4(w230) -> ()
          n185 = feedback-in #5(w224) -> ()
          n186 = case shown="False" FALSE {
            tunnel: [w244 w246] -> w232
            tunnel: w231 -> [w244 w247]
            tunnel: w213 -> [_ w245]
            frame False {
            }
            frame True {
              n187 = property class="Robot"(reference=w247, "kick_x"=w245) -> (reference out=w246:refnum<class "Robot.lvclass">)  [unwired: 1 in, 1 out]
            }
          }
          n188 = property class="PenaltyTactic"(reference=w240, "States"=w230) -> (reference out=w239:refnum<class "PenaltyTactic.lvclass">)  [unwired: 1 in, 1 out]
          n189 = property class="Robot"(reference=w232, "tactic"=tactics."PenaltyAttacker") -> (reference out=w238:refnum<class "Robot.lvclass">)  [unwired: 1 in, 1 out]
        }
      }
    }
    frame Error {
    }
  }
  "error out" <- w7
  "PenaltyTactic out" <- w5
  "Robot out" <- w3
